vi "Init.vi"(8 "error in (no error)":errorcluster, 10 "Node Reg":refnum<k20>, 11 "PropertyNode in":refnum<class "PropertyNode.lvclass">) -> (0 "error out":errorcluster, 3 "PropertyNode out":refnum<class "PropertyNode.lvclass">)   [LabVIEW 2025, in "PropertyNode.lvclass"]
uses:
  PropertyNode.lvclass
  GrowableFunctionNode.ctl
  Node/Node.lvclass
  <vilib>/xml/NI_XML.lvlib
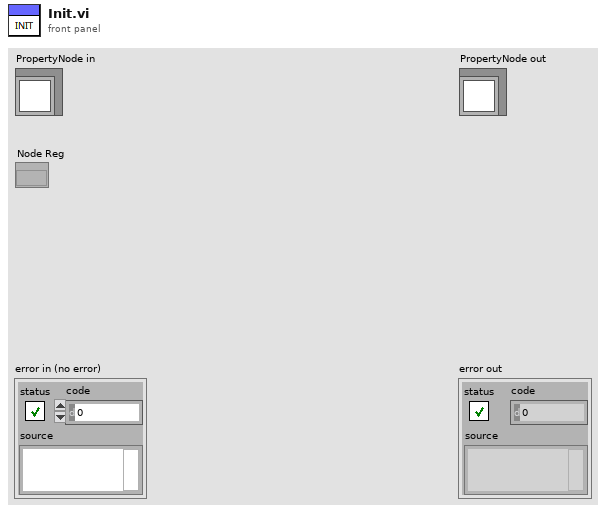
[diagram p1: front panel]
types:
  T1 = typedef "GrowableFunctionNode.ctl" = cluster{"terminalUUID":string, "Write":bool}
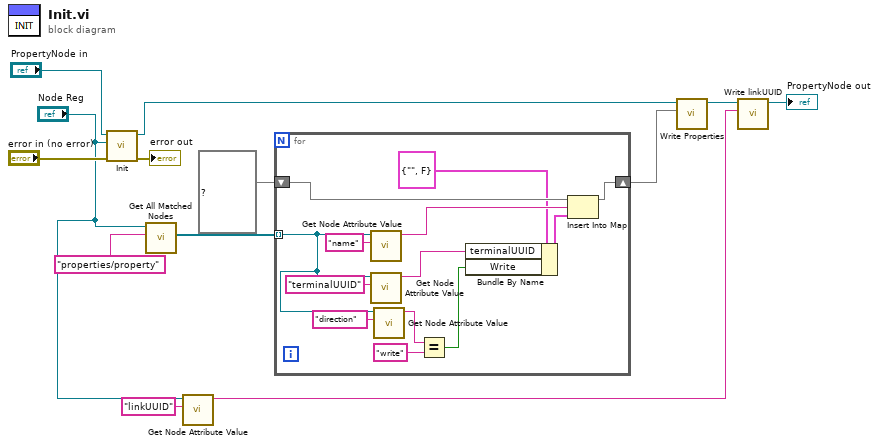
[diagram p0: block diagram]
diagram:
  n1 = call-parent "Init.vi"("error in (no error)"="error in (no error)", "Node Reg"="Node Reg", "Node in"="PropertyNode in") -> ("error out"=→"error out":errorcluster, "Node out"=w5:refnum<class "PropertyNode.lvclass">)  [unwired: 7 in]
  n2 = call <vilib>:"Get All Matched Nodes.vi"("XPath expression"="properties/property", "node in"="Node Reg") -> ("node result array"=w9:refnum<k20>[])  [unwired: 7 in, 2 out]
  n3 = call "Get Node Attribute Value.vi"("Attribute Name"="linkUUID", "Refnum in"="Node Reg") -> ("Value"=w1:string)  [unwired: 9 in]
  n4 = for {
    tunnel: w9 -> [w17] mode=indexing
    shift-right: [w22] -> w6
    shift-left: map{string, T1} {} ("Properties") -> [w23]
    n5 = call "Get Node Attribute Value.vi"("Attribute Name"="name", "Refnum in"=w17) -> ("Value"=w24:string)  [unwired: 9 in]
    n6 = call "Get Node Attribute Value.vi"("Attribute Name"="terminalUUID", "Refnum in"=w17) -> ("Value"=w19:string)  [unwired: 9 in]
    n7 = call "Get Node Attribute Value.vi"("Attribute Name"="direction", "Refnum in"=w17) -> ("Value"=w16:string)  [unwired: 9 in]
    n8 = Equal?(x=w16, y="write") -> (x = y?=w14:bool)
    n9 = Bundle By Name(cluster=T1 {"terminalUUID"="", "Write"=FALSE} ("value"), "terminalUUID"=w19, "Write"=w14) -> (w20:T1)
    n10 = Insert Into Map(map in=w23, key=w24, value=w20) -> (map out=w22:map{string, T1})  [unwired: 2 out]
  }
  n11 = call-dynamic "Write Properties.vi"("Properties"=w6, "PropertyNode in"=w5) -> ("PropertyNode out"=w8:refnum<class "PropertyNode.lvclass">)  [unwired: 8 in, 1 out]
  n12 = call-dynamic "Write linkUUID.vi"("linkUUID"=w1, "GrowableObjectFunction in"=w8) -> ("GrowableObjectFunction out"=→"PropertyNode out":refnum<class "PropertyNode.lvclass">)  [unwired: 8 in, 1 out]
